vi "Wait for Connection.vi"(8 "error in":errorcluster) -> (0 "error out":errorcluster, 3 "Cancelled":bool)   [LabVIEW 2017]
uses:
  controls/FGV DO.ctl
  99b7b577-4f86-45a1-b8ef-61e590597295.vi
panel:
  out "source":string
  in  "Cancel":bool
  # "Initialising connection to DAQ"
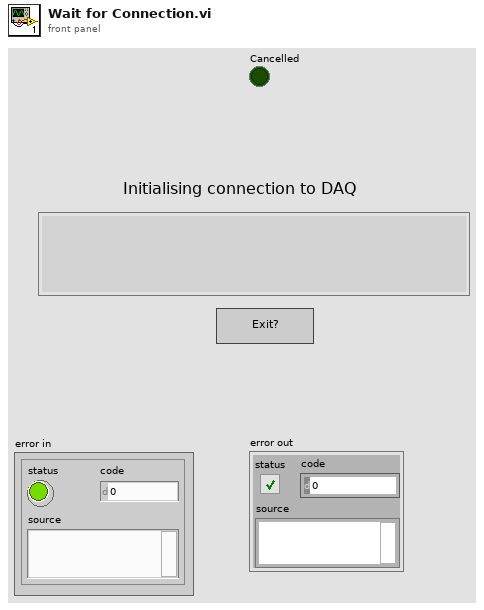
[diagram p1: front panel]
types:
  T1 = typedef "FGV DO.ctl" = enum16{"Initialize", "Clamping", "Load CYL", "Contactors", "Clear Tasks"}
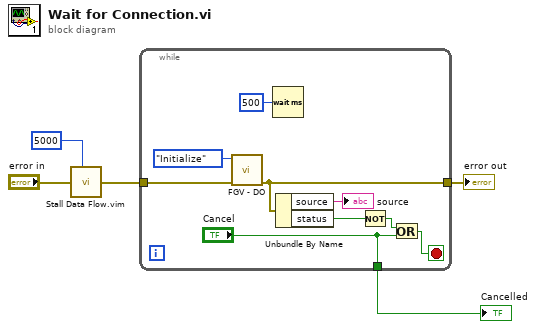
[diagram p0: block diagram]
diagram:
  n1 = call "Stall Data Flow.vim"("value in"="error in", "milliseconds to wait"=u32 5000) -> ("value out"=w3:errorcluster)  [unwired: 1 out]
  n2 = while {
    tunnel: [w10] -> w5
    tunnel: w3 -> [w11]
    tunnel: ["Cancel"] -> w1
    stop <- w12 stop-if-true
    n3 = call "FGV - DO.vi"("error in"=w11, "State"=FGV_DO."Initialize") -> ("error out"=w10:errorcluster)  [unwired: 9 in]
    n4 = Wait (ms)(milliseconds to wait=u32 500) -> ()  [unwired: 1 out]
    n5 = Unbundle By Name(w10) -> ("source"=→"source":string, "status"=w9:bool)
    n6 = Not(x=w9) -> (.not. x?=w8:bool)
    n7 = Or(x=w8, y="Cancel") -> (x .or. y?=w12:bool)
  }
  "error out" <- w5
  "Cancelled" <- w1
